vi "GetText.vi"(8 "error in":errorcluster, 11 "WaveformAcq editor node in":refnum<class "WaveformAcq editor node.lvclass">) -> (0 "error out":errorcluster, 1 "additional text":string, 2 "text":string, 3 "WaveformAcq editor node out":refnum<class "WaveformAcq editor node.lvclass">, 4 "glyph":string)   [LabVIEW 2017, in "WaveformAcq editor node.lvclass"]
uses:
  WaveformAcq editor node.lvclass
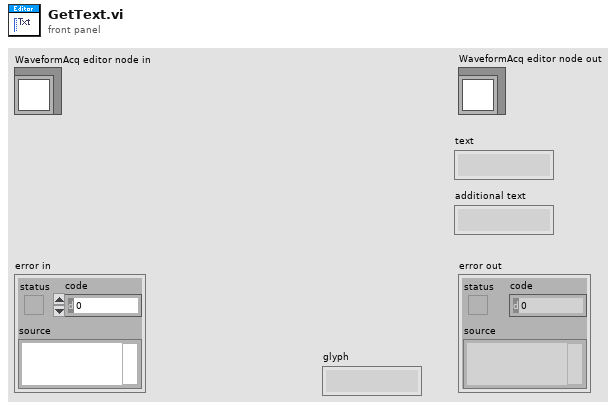
[diagram p1: front panel]
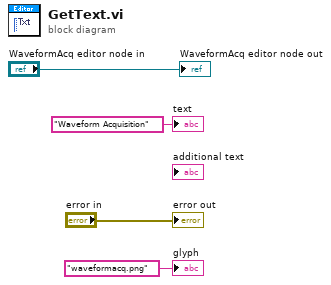
[diagram p0: block diagram]
diagram:
  "error out" <- "error in"
  "WaveformAcq editor node out" <- "WaveformAcq editor node in"
  "text" <- "Waveform Acquisition" ("text")
  "glyph" <- "waveformacq.png" ("glyph")
